vi "Chad Magic Voodoo 4.vi"() -> ()   [LabVIEW 2016]
panel:
  in  "Automatic Wire\n Feed not to Exceed":dbl=1.4
  in  "Add Wire Feed... (%)":dbl=4.0
  in  "For Every... (mm)":dbl=0.2
  out "W trigger Y":dbl
  out "C trigger Y":dbl
  out "R trigger Y":dbl
  in  "Window Bead Trigger heights":dbl[](array[numeric])
  in  "Robot Bead Trigger heights":dbl[](array[numeric])
  in  "Center Bead Trigger heights":dbl[](array[numeric])
  out "Shutter Open":bool
  in  "base path":path=path "C:/Users/Mark/Desktop/BeadScan"
  in  "Write Code":bool
  out "Bead3 Size":i32
  out "Bead2 Size":i32
  out "Bead1 Size":i32
  in  "Tab Control":T1(tab)
  in  "Mark Target Bead Height":bool
  out "All Beads":cluster{dbl[], dbl[]}[](graph)
  out "Target Bead Height":dbl
  in  "Set Correction C":bool
  in  "Set Trigger Offset":dbl
  in  "Center Bead Corrections":dbl[](array[numeric])
  in  "Center Bead Trigger Positions":dbl[](array[numeric])
  out "Center Bead #1":cluster{dbl[], dbl[]}[](graph)
  out "Center Bead Trigger":dbl
  in  "Set Trigger Center":bool
  in  "Undo":bool
  out "Difference From Bead Height Setpoint C":dbl
  out "Recommended % Change\n in Wire Feed C":dbl
  in  "Set Correction R":bool
  in  "Set Trigger Offset 2":dbl
  out "Robot Bead #2":cluster{dbl[], dbl[]}[](graph)
  in  "Robot Bead Trigger Positions":dbl[](array[numeric])
  in  "Robot Bead Corrections":dbl[](array[numeric])
  out "Robot Bead Trigger":dbl
  in  "Set Trigger Robot":bool
  in  "Undo":bool
  out "Difference From Bead Height Setpoint R":dbl
  out "Recommended % Change\n in Wire Feed R":dbl
  in  "Set Correction W":bool
  in  "Set Trigger Offset 3":dbl
  out "Window Bead #3":cluster{dbl[], dbl[]}[](graph)
  in  "Window Bead Trigger Positions":dbl[](array[numeric])
  in  "Window Bead Corrections":dbl[](array[numeric])
  out "Window Bead Trigger":dbl
  in  "Set Trigger Window":bool
  in  "Undo":bool
  out "Difference From Bead Height Setpoint W":dbl
  out "Recommended % Change\n in Wire Feed W":dbl
  in  "stop":bool
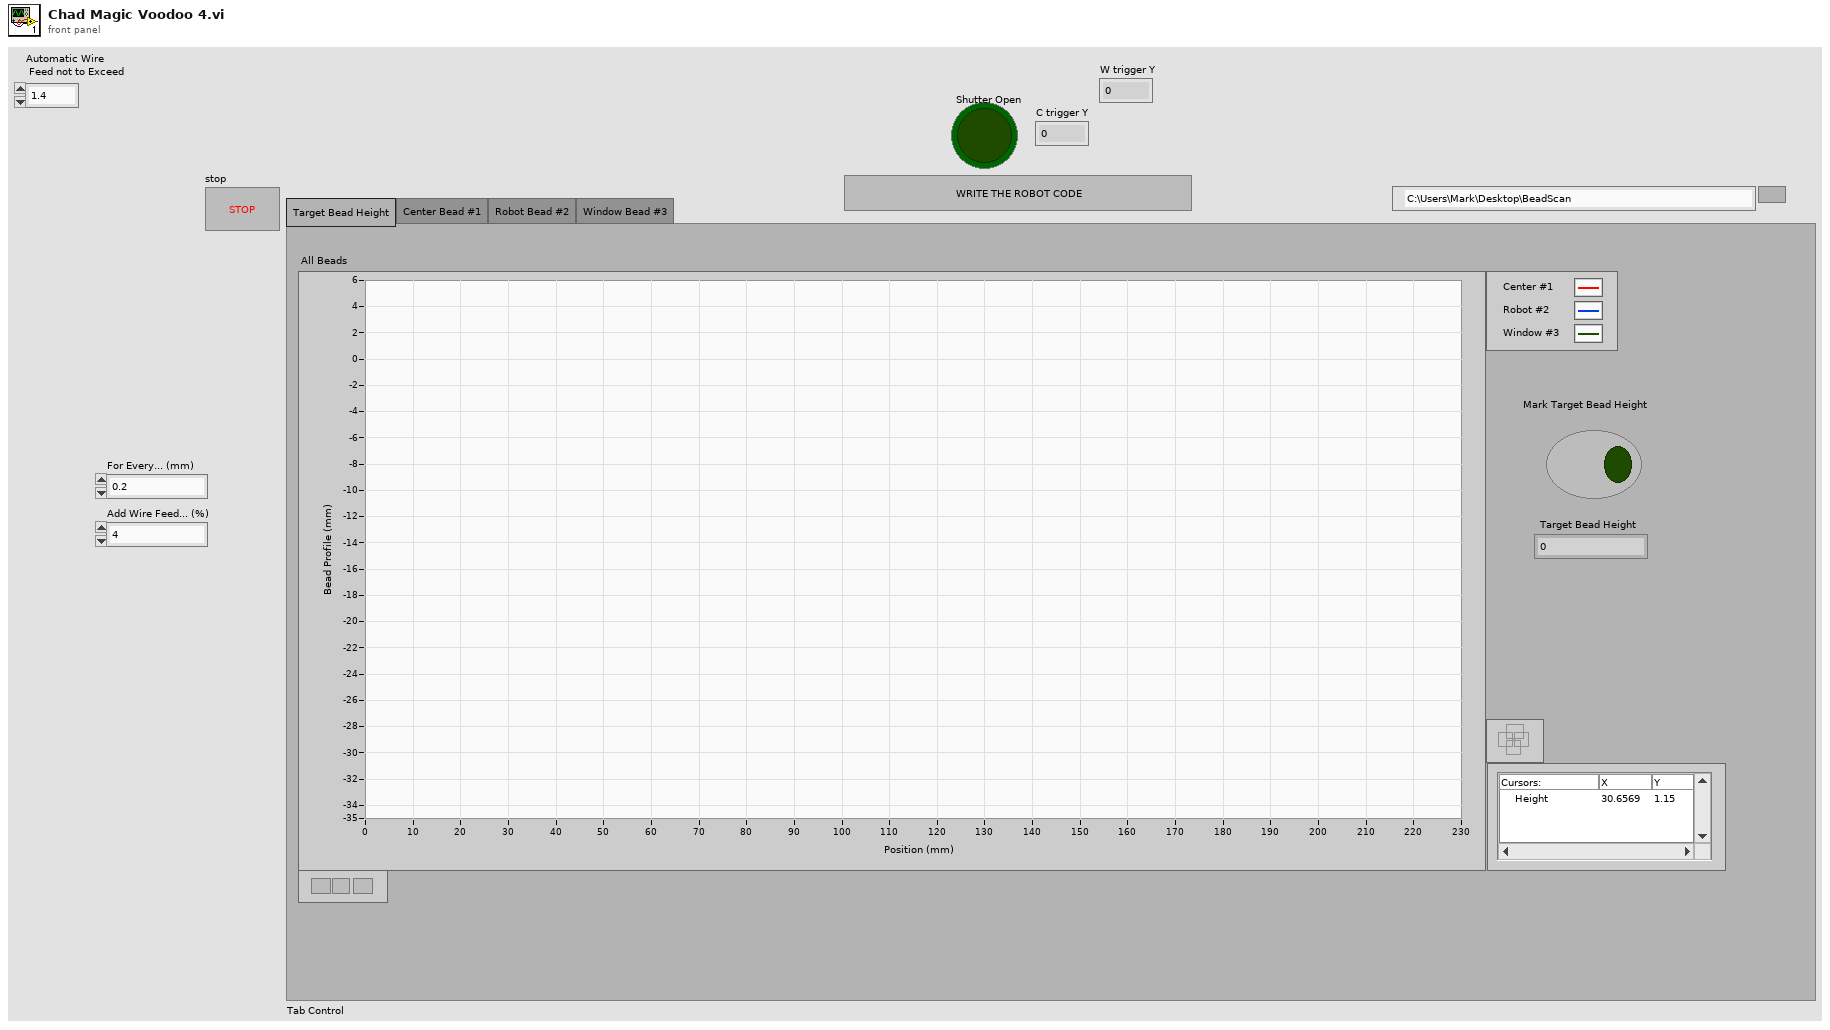
[diagram p1: front panel]
types:
  T1 = enum32{"Target Bead Height", "Center Bead #1", "Robot Bead #2", "Window Bead #3"}
  T2 = enum16{"open", "replace", "create", "open or create", "replace or create", "replace or create with confirmation"}
  T3 = cluster{"[0]":cluster{dbl[], dbl[]}, "[1]":cluster{dbl[], dbl[]}, "[2]":cluster{dbl[], dbl[]}}
  T4 = cluster{dbl[], "Center Bead Trigger heights":dbl[]}
  T5 = cluster{dbl[], "Window Bead Trigger heights":dbl[]}
  T6 = cluster{dbl[], "Robot Bead Trigger heights":dbl[]}
  T7 = cluster{dbl[], "Center Bead Trigger heights":dbl[]}[]
  T8 = cluster{dbl[], "Robot Bead Trigger heights":dbl[]}[]
  T9 = cluster{dbl[], "Window Bead Trigger heights":dbl[]}[]
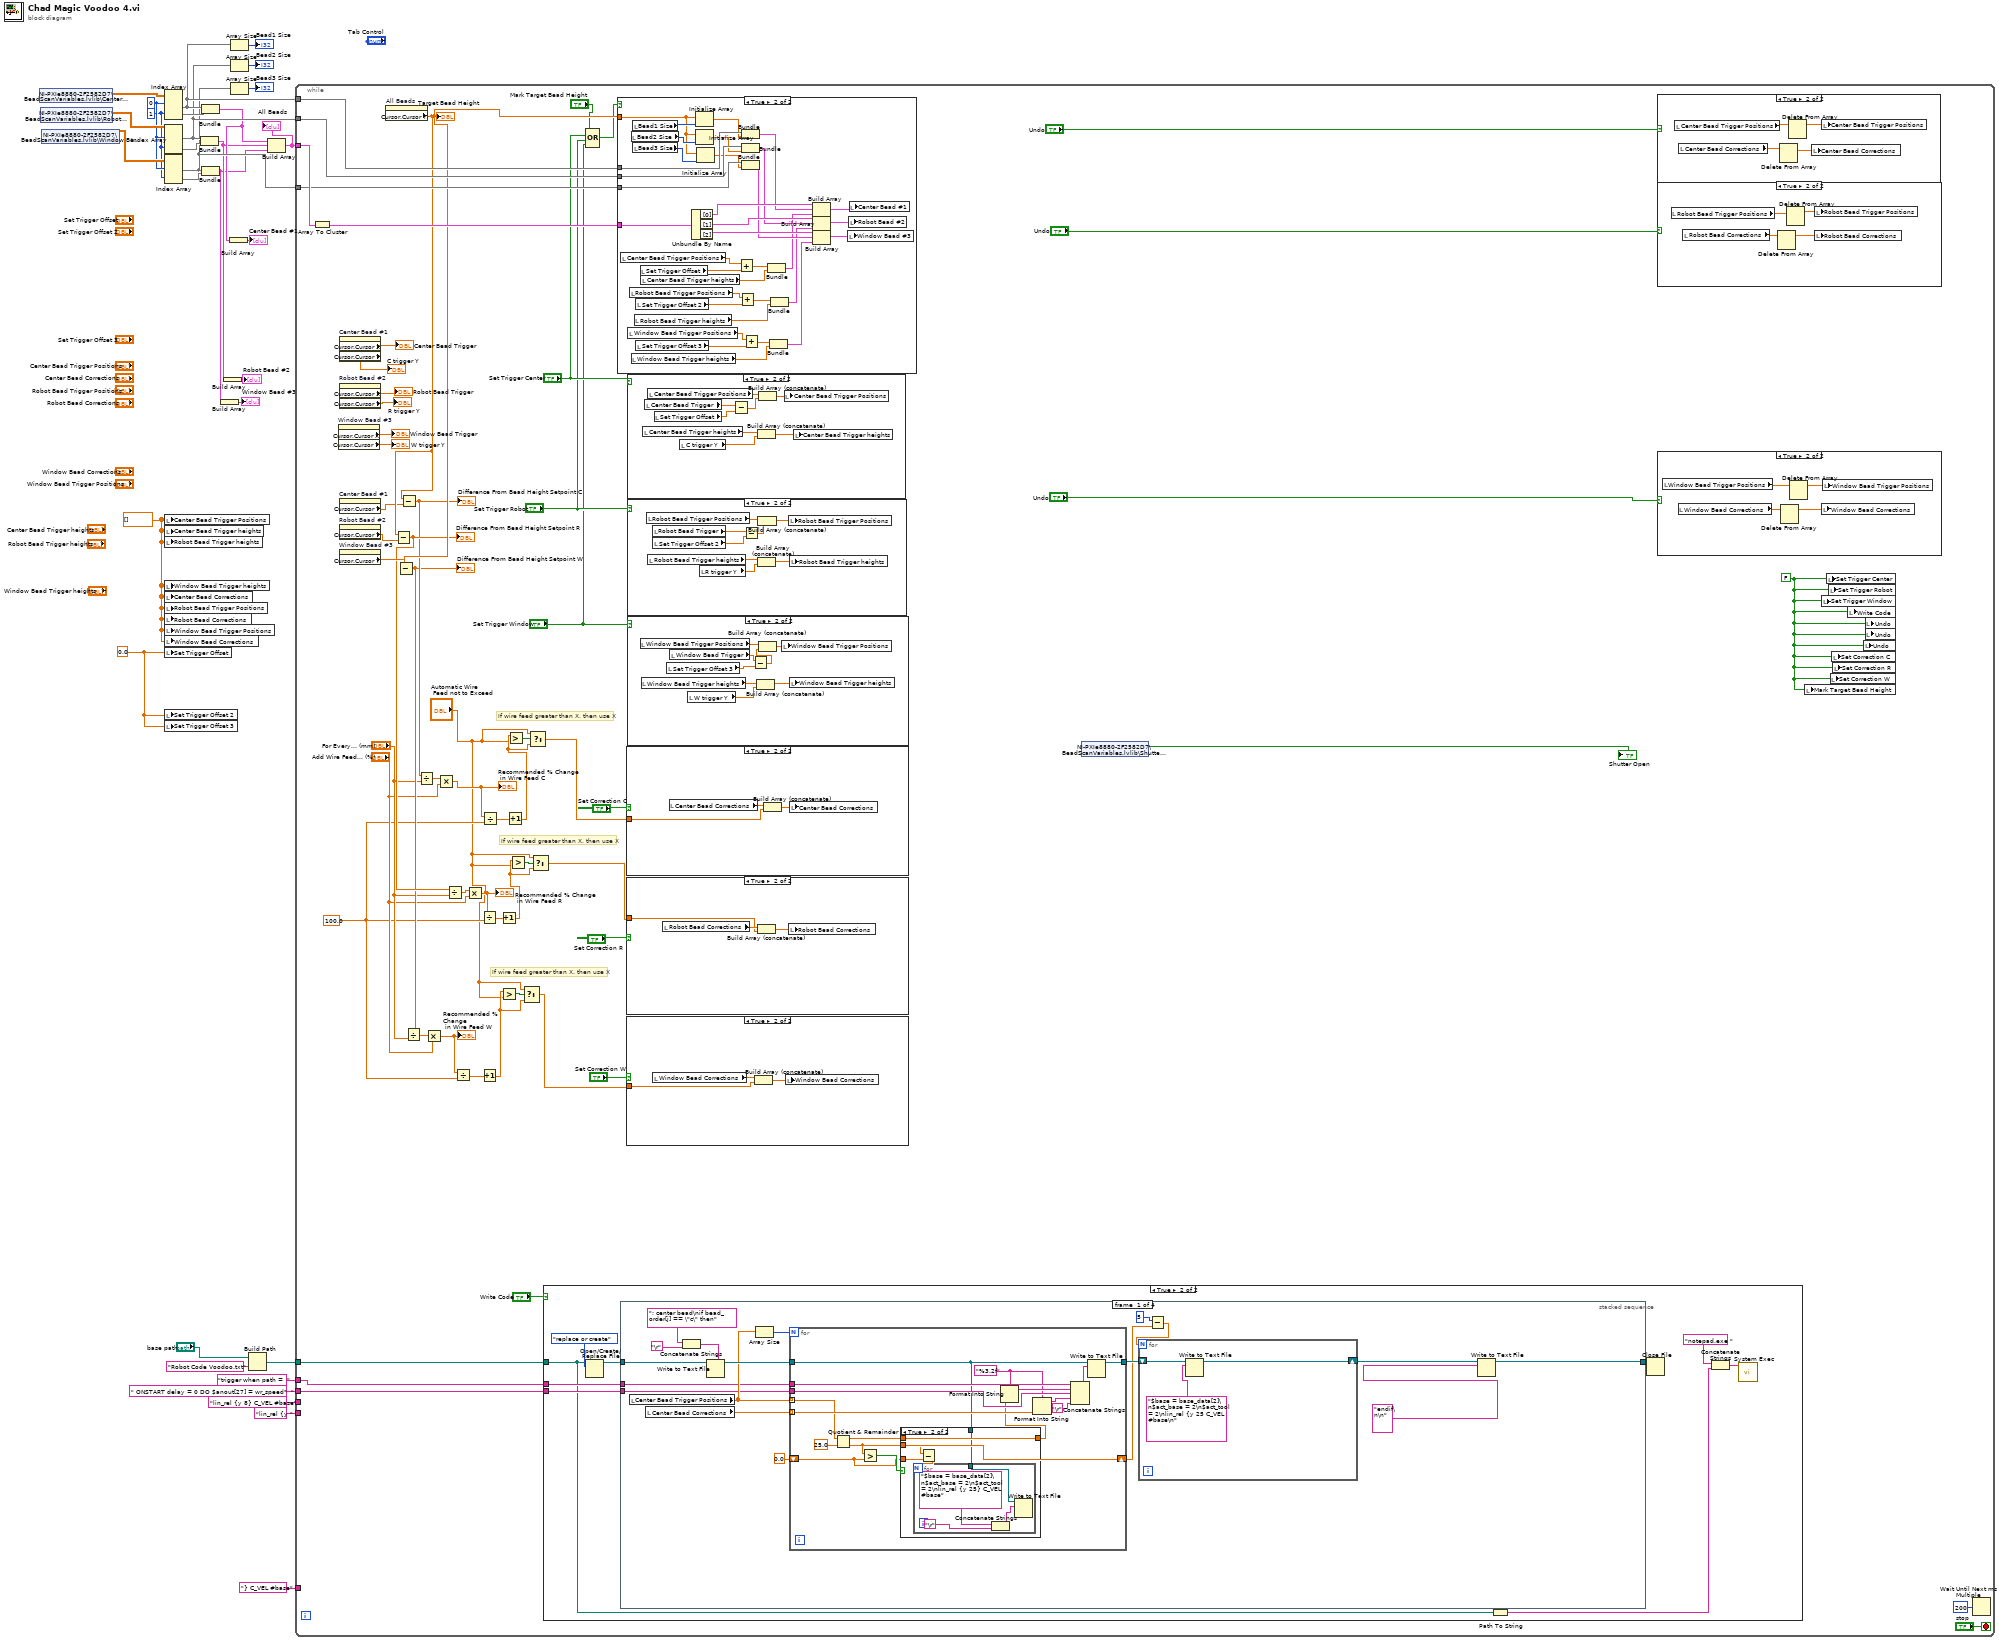
[diagram p0: block diagram]
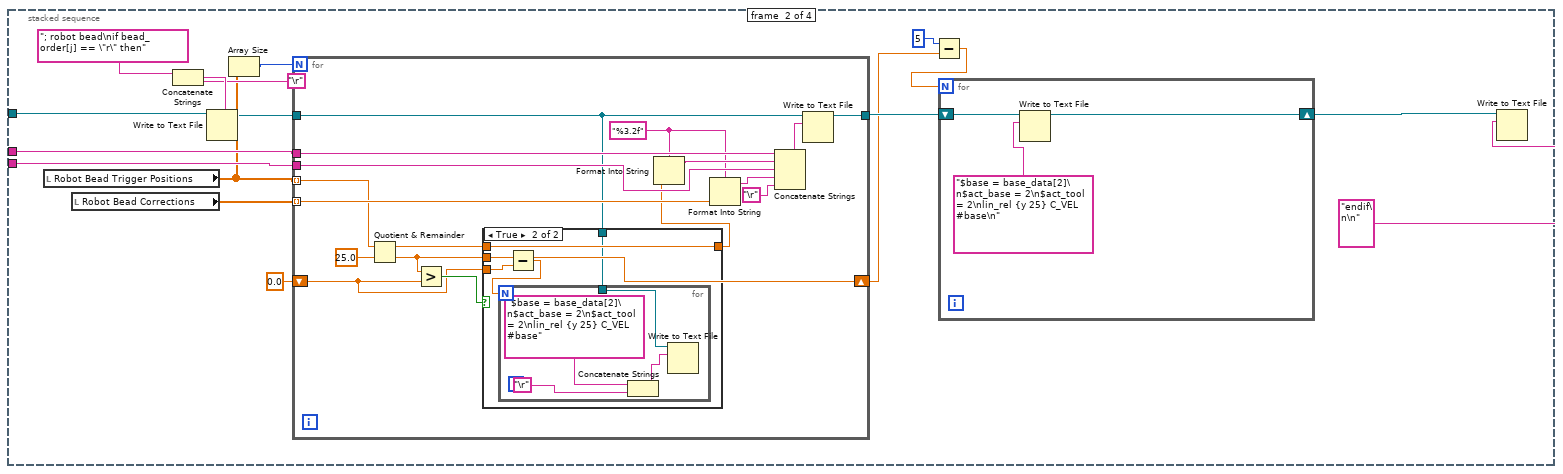
[diagram p7: hidden frame]
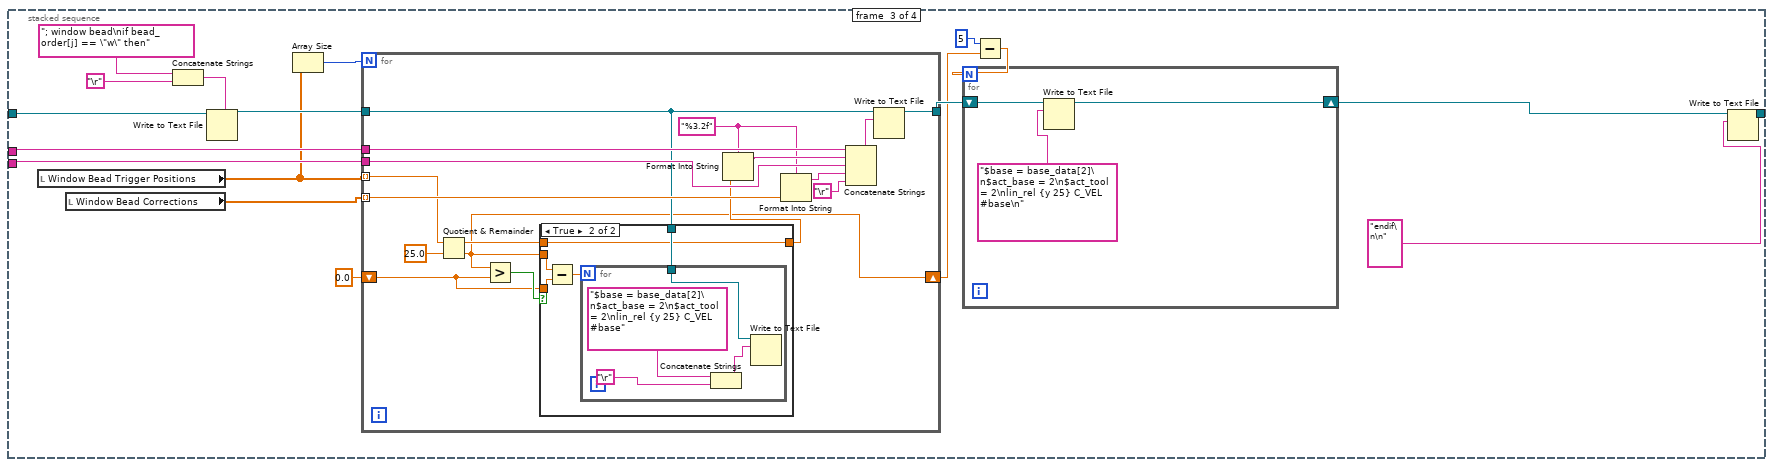
[diagram p9: hidden frame]
diagram:
  w2 = 0.0
  w1 = dbl[] []
  w26 = 1 ("index (row)")
  w27 = 0 ("index (row)")
  n1 = shared-variable "NI-PXIe8880-2F2582D7\\BeadScanVariables.lvlib\\Center Bead #1"() -> (w31:dbl[][])  [unwired: 1 in, 1 out]
  n2 = shared-variable "NI-PXIe8880-2F2582D7\\BeadScanVariables.lvlib\\Robot Bead #2"() -> (w29:dbl[][])  [unwired: 1 in, 1 out]
  n3 = shared-variable "NI-PXIe8880-2F2582D7\\BeadScanVariables.lvlib\\Window Bead #3"() -> (w28:dbl[][])  [unwired: 1 in, 1 out]
  n4 = Index Array(array=w31, index (row) #1=w27, index (row) #2=w26) -> (element #1=w19:dbl[], element #2=w30:dbl[])  [unwired: 2 in]
  n5 = Index Array(array=w29, index (row) #1=w27, index (row) #2=w26) -> (element #1=w18:dbl[], element #2=w25:dbl[])  [unwired: 2 in]
  n6 = Index Array(array=w28, index (row) #1=w27, index (row) #2=w26) -> (element #1=w17:dbl[], element #2=w24:dbl[])  [unwired: 2 in]
  n7 = local write "Center Bead Trigger Positions"(w1) -> ()
  n8 = local write "Center Bead Trigger heights"(w1) -> ()
  n9 = local write "Robot Bead Trigger heights"(w1) -> ()
  n10 = local write "Window Bead Trigger heights"(w1) -> ()
  n11 = local write "Center Bead Corrections"(w1) -> ()
  n12 = local write "Robot Bead Trigger Positions"(w1) -> ()
  n13 = local write "Robot Bead Corrections"(w1) -> ()
  n14 = local write "Window Bead Trigger Positions"(w1) -> ()
  n15 = local write "Window Bead Corrections"(w1) -> ()
  n16 = local write "Set Trigger Offset"(w2) -> ()
  n17 = local write "Set Trigger Offset 2"(w2) -> ()
  n18 = local write "Set Trigger Offset 3"(w2) -> ()
  n19 = Bundle(w18, w25) -> (w14:cluster{dbl[], dbl[]})  [unwired: 1 in]
  n20 = Bundle(w19, w30) -> (w15:cluster{dbl[], dbl[]})  [unwired: 1 in]
  n21 = Bundle(w17, w24) -> (w11:cluster{dbl[], dbl[]})  [unwired: 1 in]
  n22 = Build Array(w11) -> (→"Window Bead #3":cluster{dbl[], dbl[]}[])
  n23 = Build Array(w14) -> (→"Robot Bead #2":cluster{dbl[], dbl[]}[])
  n24 = Build Array(w15) -> (→"Center Bead #1":cluster{dbl[], dbl[]}[])
  n25 = Array Size(array=w19) -> (size(s)=→"Bead1 Size":i32)
  n26 = Array Size(array=w18) -> (size(s)=→"Bead2 Size":i32)
  n27 = Array Size(array=w17) -> (size(s)=→"Bead3 Size":i32)
  n28 = Build Path(base path="base path", name or relative path="Robot Code Voodoo.txt") -> (appended path=w8:path)
  n29 = Build Array(w15, w14, w11) -> (w20:cluster{dbl[], dbl[]}[])
  "All Beads" <- w20
  n30 = while {
    tunnel: w20 -> [w87]
    tunnel: w19 -> [w85]
    tunnel: w18 -> [w84]
    tunnel: w17 -> [w83]
    tunnel: w8 -> [w78]
    tunnel: "trigger when path =  " -> [w77]
    tunnel: " ONSTART delay = 0 DO $anout[27] = wr_speed*  " -> [w76]
    tunnel: "lin_rel {y 8} C_VEL #base" -> [_]
    tunnel: "lin_rel {y " -> [_]
    tunnel: "} C_VEL #base" -> [_]
    stop <- "stop" stop-if-true
    w46 = 100.0 ("y")
    w42 = FALSE
    # "If wire feed greater than X, then use X"
    # "If wire feed greater than X, then use X"
    # "If wire feed greater than X, then use X"
    n31 = Array To Cluster(array=w87) -> (cluster=w86:T3)
    n32 = property on="Window Bead #3" class="XYGraph (strict)"() -> ("Cursor.Cursor X"=→"Window Bead Trigger":dbl, "Cursor.Cursor Y"=→"W trigger Y":dbl)  [unwired: 2 in, 2 out]
    n33 = property on="Center Bead #1" class="XYGraph (strict)"() -> ("Cursor.Cursor X"=→"Center Bead Trigger":dbl, "Cursor.Cursor Y"=→"C trigger Y":dbl)  [unwired: 2 in, 2 out]
    n34 = property on="Robot Bead #2" class="XYGraph (strict)"() -> ("Cursor.Cursor X"=→"Robot Bead Trigger":dbl, "Cursor.Cursor Y"=→"R trigger Y":dbl)  [unwired: 2 in, 2 out]
    n35 = property on="Center Bead #1" class="XYGraph (strict)"() -> ("Cursor.Cursor Y"=w72:dbl)  [unwired: 2 in, 2 out]
    n36 = property on="Robot Bead #2" class="XYGraph (strict)"() -> ("Cursor.Cursor Y"=w71:dbl)  [unwired: 2 in, 2 out]
    n37 = property on="Window Bead #3" class="XYGraph (strict)"() -> ("Cursor.Cursor Y"=w70:dbl)  [unwired: 2 in, 2 out]
    n38 = property on="All Beads" class="XYGraph (strict)"() -> ("Cursor.Cursor Y"=w73:dbl)  [unwired: 2 in, 2 out]
    "Target Bead Height" <- w73
    n39 = Subtract(x=w73, y=w71) -> (x-y=w58:dbl)
    "Difference From Bead Height Setpoint R" <- w58
    n40 = Subtract(x=w73, y=w70) -> (x-y=w55:dbl)
    "Difference From Bead Height Setpoint W" <- w55
    n41 = Subtract(x=w73, y=w72) -> (x-y=w56:dbl)
    "Difference From Bead Height Setpoint C" <- w56
    n42 = Divide(x=w55, y="For Every... (mm)") -> (x/y=w59:dbl)
    n43 = Divide(x=w56, y="For Every... (mm)") -> (x/y=w57:dbl)
    n44 = Multiply(x=w59, y="Add Wire Feed... (%)") -> (x*y=w47:dbl)
    "Recommended % Change\n in Wire Feed W" <- w47
    n45 = Multiply(x=w57, y="Add Wire Feed... (%)") -> (x*y=w48:dbl)
    "Recommended % Change\n in Wire Feed C" <- w48
    n46 = Divide(x=w58, y="For Every... (mm)") -> (x/y=w60:dbl)
    n47 = Divide(x=w47, y=w46) -> (x/y=w43:dbl)
    n48 = Multiply(x=w60, y="Add Wire Feed... (%)") -> (x*y=w49:dbl)
    "Recommended % Change\n in Wire Feed R" <- w49
    n49 = Divide(x=w49, y=w46) -> (x/y=w45:dbl)
    n50 = Increment(x=w43) -> (x+1=w35:dbl)
    n51 = Divide(x=w48, y=w46) -> (x/y=w44:dbl)
    n52 = Increment(x=w45) -> (x+1=w33:dbl)
    n53 = Greater?(x=w35, y="Automatic Wire\n Feed not to Exceed") -> (0:w37:bool)
    n54 = Increment(x=w44) -> (x+1=w39:dbl)
    n55 = Greater?(x=w39, y="Automatic Wire\n Feed not to Exceed") -> (0:w41:bool)
    n56 = Greater?(x=w33, y="Automatic Wire\n Feed not to Exceed") -> (0:w38:bool)
    n57 = Select(t="Automatic Wire\n Feed not to Exceed", s=w37, f=w35) -> (s? t:f=w36:dbl)
    n58 = Select(t="Automatic Wire\n Feed not to Exceed", s=w41, f=w39) -> (s? t:f=w40:dbl)
    n59 = Select(t="Automatic Wire\n Feed not to Exceed", s=w38, f=w33) -> (s? t:f=w34:dbl)
    n60 = case shown="True" "Write Code" {
      tunnel: w78 -> [_ w100]
      tunnel: w77 -> [_ w107]
      tunnel: w76 -> [_ w106]
      frame False {
      }
      frame True {
        n61 = Open/Create/Replace File(file path (use dialog)=w100, operation (0:open)=T2."replace or create") -> (refnum out=w108:refnum<file>)  [unwired: 4 in, 2 out]
        n62 = stacked-sequence {
          tunnel: w108 -> [w123 w171 w218 _]
          tunnel: w107 -> [w118 w168 w213 _]
          tunnel: w106 -> [w117 w167 w212 _]
          tunnel: [w114 _ _ _] -> w105
          frame #0 {
            n63 = local read "Center Bead Trigger Positions"() -> (w120:dbl[])
            n64 = local read "Center Bead Corrections"() -> (w119:dbl[])
            n65 = Concatenate Strings("; center bead\nif bead_order[j] == \"c\" then", "\r") -> (w124:string)
            n66 = Write to Text File(file (use dialog)=w123, text=w124) -> (refnum out=w122:refnum<file>)  [unwired: 2 in, 2 out]
            n67 = Array Size(array=w120) -> (size(s)=w121:i32)
            n68 = for {
              N: w121 -> [_]
              tunnel: w122 -> [w132]
              tunnel: w120 -> [w137] mode=indexing
              tunnel: w119 -> [w142] mode=indexing
              tunnel: w118 -> [w146]
              tunnel: w117 -> [w143]
              tunnel: [w140] -> w115
              shift-right: [w131] -> w110
              shift-left: 0.0 -> [w130]
              w139 = "%3.2f" ("format string")
              n69 = Quotient & Remainder(x=w137, y=25.0) -> (x-y*floor(x/y)=w134:dbl, floor(x/y)=w131:dbl)
              n70 = Greater?(x=w131, y=w130) -> (0:w135:bool)
              n71 = case shown="True" w135 {
                tunnel: w134 -> [w147 w152]
                tunnel: [w147 w152] -> w133
                tunnel: w132 -> [_ w151]
                tunnel: w131 -> [_ w150]
                tunnel: w130 -> [_ w149]
                frame False {
                }
                frame True {
                  n72 = Subtract(x=w150, y=w149) -> (x-y=w148:dbl)
                  n73 = for {
                    N: w148 -> [_]
                    tunnel: w151 -> [w156]
                    n74 = Concatenate Strings("$base = base_data[2]\n$act_base = 2\n$act_tool = 2\nlin_rel {y 25} C_VEL #base", "\r") -> (w153:string)
                    n75 = Write to Text File(file (use dialog)=w156, text=w153) -> ()  [unwired: 2 in, 3 out]
                  }
                }
              }
              n76 = Format Into String(format string=w139, w133) -> (resulting string=w145:string)  [unwired: 2 in, 1 out]
              n77 = Format Into String(format string=w139, w142) -> (resulting string=w141:string)  [unwired: 2 in, 1 out]
              n78 = Concatenate Strings(w146, w145, w143, w141, "\r") -> (w144:string)
              n79 = Write to Text File(file (use dialog)=w132, text=w144) -> (refnum out=w140:refnum<file>)  [unwired: 2 in, 2 out]
            }
            n80 = Subtract(x=5, y=w110) -> (x-y=w109:dbl)
            n81 = for {
              N: w109 -> [_]
              shift-right: [w127] -> w113
              shift-left: w115 -> [w129]
              n82 = Write to Text File(file (use dialog)=w129, text="$base = base_data[2]\n$act_base = 2\n$act_tool = 2\nlin_rel {y 25 C_VEL #base\n") -> (refnum out=w127:refnum<file>)  [unwired: 2 in, 2 out]
            }
            n83 = Write to Text File(file (use dialog)=w113, text="endif\n\n") -> (refnum out=w114:refnum<file>)  [unwired: 2 in, 2 out]
          }
          frame #1 {
            n84 = local read "Robot Bead Trigger Positions"() -> (w166:dbl[])
            n85 = local read "Robot Bead Corrections"() -> (w165:dbl[])
            n86 = Concatenate Strings("; robot bead\nif bead_order[j] == \"r\" then", "\r") -> (w172:string)
            n87 = Write to Text File(file (use dialog)=w171, text=w172) -> (refnum out=w164:refnum<file>)  [unwired: 2 in, 2 out]
            n88 = Array Size(array=w166) -> (size(s)=w163:i32)
            n89 = for {
              N: w163 -> [_]
              tunnel: w164 -> [w179]
              tunnel: w166 -> [w184] mode=indexing
              tunnel: w165 -> [w189] mode=indexing
              tunnel: w168 -> [w193]
              tunnel: w167 -> [w190]
              tunnel: [w187] -> w158
              shift-right: [w178] -> w157
              shift-left: 0.0 -> [w177]
              w186 = "%3.2f" ("format string")
              n90 = Quotient & Remainder(x=w184, y=25.0) -> (x-y*floor(x/y)=w181:dbl, floor(x/y)=w178:dbl)
              n91 = Greater?(x=w178, y=w177) -> (0:w182:bool)
              n92 = case shown="True" w182 {
                tunnel: w181 -> [w194 w199]
                tunnel: [w194 w199] -> w180
                tunnel: w179 -> [_ w198]
                tunnel: w178 -> [_ w197]
                tunnel: w177 -> [_ w196]
                frame False {
                }
                frame True {
                  n93 = Subtract(x=w197, y=w196) -> (x-y=w195:dbl)
                  n94 = for {
                    N: w195 -> [_]
                    tunnel: w198 -> [w203]
                    n95 = Concatenate Strings("$base = base_data[2]\n$act_base = 2\n$act_tool = 2\nlin_rel {y 25} C_VEL #base", "\r") -> (w200:string)
                    n96 = Write to Text File(file (use dialog)=w203, text=w200) -> ()  [unwired: 2 in, 3 out]
                  }
                }
              }
              n97 = Format Into String(format string=w186, w180) -> (resulting string=w192:string)  [unwired: 2 in, 1 out]
              n98 = Format Into String(format string=w186, w189) -> (resulting string=w188:string)  [unwired: 2 in, 1 out]
              n99 = Concatenate Strings(w193, w192, w190, w188, "\r") -> (w191:string)
              n100 = Write to Text File(file (use dialog)=w179, text=w191) -> (refnum out=w187:refnum<file>)  [unwired: 2 in, 2 out]
            }
            n101 = Subtract(x=5, y=w157) -> (x-y=w159:dbl)
            n102 = for {
              N: w159 -> [_]
              shift-right: [w174] -> w162
              shift-left: w158 -> [w176]
              n103 = Write to Text File(file (use dialog)=w176, text="$base = base_data[2]\n$act_base = 2\n$act_tool = 2\nlin_rel {y 25} C_VEL #base\n") -> (refnum out=w174:refnum<file>)  [unwired: 2 in, 2 out]
            }
            n104 = Write to Text File(file (use dialog)=w162, text="endif\n\n") -> ()  [unwired: 2 in, 3 out]
          }
          frame #2 {
            n105 = local read "Window Bead Trigger Positions"() -> (w211:dbl[])
            n106 = local read "Window Bead Corrections"() -> (w210:dbl[])
            n107 = Concatenate Strings("; window bead\nif bead_order[j] == \"w\" then", "\r") -> (w219:string)
            n108 = Write to Text File(file (use dialog)=w218, text=w219) -> (refnum out=w214:refnum<file>)  [unwired: 2 in, 2 out]
            n109 = Array Size(array=w211) -> (size(s)=w215:i32)
            n110 = for {
              N: w215 -> [_]
              tunnel: w214 -> [w226]
              tunnel: w211 -> [w231] mode=indexing
              tunnel: w210 -> [w236] mode=indexing
              tunnel: w213 -> [w240]
              tunnel: w212 -> [w237]
              tunnel: [w234] -> w205
              shift-right: [w225] -> w204
              shift-left: 0.0 -> [w224]
              w233 = "%3.2f" ("format string")
              n111 = Quotient & Remainder(x=w231, y=25.0) -> (x-y*floor(x/y)=w228:dbl, floor(x/y)=w225:dbl)
              n112 = Greater?(x=w225, y=w224) -> (0:w229:bool)
              n113 = case shown="True" w229 {
                tunnel: w228 -> [w241 w245]
                tunnel: [w241 w245] -> w227
                tunnel: w226 -> [_ w246]
                tunnel: w225 -> [_ w243]
                tunnel: w224 -> [_ w242]
                frame False {
                }
                frame True {
                  n114 = Subtract(x=w243, y=w242) -> (x-y=w244:dbl)
                  n115 = for {
                    N: w244 -> [_]
                    tunnel: w246 -> [w250]
                    n116 = Concatenate Strings("$base = base_data[2]\n$act_base = 2\n$act_tool = 2\nlin_rel {y 25} C_VEL #base", "\r") -> (w247:string)
                    n117 = Write to Text File(file (use dialog)=w250, text=w247) -> ()  [unwired: 2 in, 3 out]
                  }
                }
              }
              n118 = Format Into String(format string=w233, w227) -> (resulting string=w239:string)  [unwired: 2 in, 1 out]
              n119 = Format Into String(format string=w233, w236) -> (resulting string=w235:string)  [unwired: 2 in, 1 out]
              n120 = Concatenate Strings(w240, w239, w237, w235, "\r") -> (w238:string)
              n121 = Write to Text File(file (use dialog)=w226, text=w238) -> (refnum out=w234:refnum<file>)  [unwired: 2 in, 2 out]
            }
            n122 = Subtract(x=5, y=w204) -> (x-y=w206:dbl)
            n123 = for {
              N: w206 -> [_]
              shift-right: [w221] -> w209
              shift-left: w205 -> [w223]
              n124 = Write to Text File(file (use dialog)=w223, text="$base = base_data[2]\n$act_base = 2\n$act_tool = 2\nlin_rel {y 25} C_VEL #base\n") -> (refnum out=w221:refnum<file>)  [unwired: 2 in, 2 out]
            }
            n125 = Write to Text File(file (use dialog)=w209, text="endif\n\n") -> ()  [unwired: 2 in, 3 out]
          }
          frame #3 {
          }
        }
        n126 = Path To String(path=w100) -> (string=w101:string)
        n127 = Close File(refnum=w105) -> ()  [unwired: 1 in, 2 out]
        n128 = Concatenate Strings("notepad.exe " ("command line"), w101) -> (w103:string)
        n129 = call <vilib>:"System Exec.vi"("command line"=w103) -> ()  [unwired: 7 in, 4 out]
      }
    }
    n130 = Compound Arithmetic op=OR("Mark Target Bead Height", "Set Trigger Center", "Set Trigger Robot", "Set Trigger Window") -> (w64:bool)
    n131 = case shown="True" w64 {
      tunnel: w73 -> [_ w319]
      tunnel: w86 -> [_ w317]
      tunnel: w85 -> [_ w316]
      tunnel: w84 -> [_ w314]
      tunnel: w83 -> [_ w313]
      frame False {
      }
      frame True {
        n132 = local read "Center Bead Trigger Positions"() -> (w297:dbl[])
        n133 = local read "Window Bead Trigger Positions"() -> (w291:dbl[])
        n134 = local read "Robot Bead Trigger Positions"() -> (w294:dbl[])
        n135 = local read "Bead2 Size"() -> (w320:i32)
        n136 = local read "Window Bead Trigger heights"() -> (w290:dbl[])
        n137 = local read "Bead1 Size"() -> (w321:i32)
        n138 = local read "Bead3 Size"() -> (w318:i32)
        n139 = local read "Robot Bead Trigger heights"() -> (w292:dbl[])
        n140 = local read "Set Trigger Offset 2"() -> (w300:dbl)
        n141 = local read "Set Trigger Offset 3"() -> (w299:dbl)
        n142 = local read "Set Trigger Offset"() -> (w301:dbl)
        n143 = local read "Center Bead Trigger heights"() -> (w295:dbl[])
        n144 = Unbundle By Name(w317) -> ("[0]"=w310:cluster{dbl[], dbl[]}, "[1]"=w308:cluster{dbl[], dbl[]}, "[2]"=w306:cluster{dbl[], dbl[]})
        n145 = Initialize Array(w319, w321) -> (w315:dbl[])
        n146 = Initialize Array(w319, w320) -> (w311:dbl[])
        n147 = Initialize Array(w319, w318) -> (w312:dbl[])
        n148 = Add(x=w297, y=w301) -> (x+y=w296:dbl[])
        n149 = Add(x=w294, y=w300) -> (x+y=w293:dbl[])
        n150 = Bundle(w316, w315) -> (w309:cluster{dbl[], dbl[]})  [unwired: 1 in]
        n151 = Bundle(w314, w311) -> (w307:cluster{dbl[], dbl[]})  [unwired: 1 in]
        n152 = Bundle(w313, w312) -> (w305:cluster{dbl[], dbl[]})  [unwired: 1 in]
        n153 = Add(x=w291, y=w299) -> (x+y=w298:dbl[])
        n154 = Bundle(w296, "Center Bead Trigger heights"=w295) -> (w289:T4)  [unwired: 1 in]
        n155 = Bundle(w298, "Window Bead Trigger heights"=w290) -> (w287:T5)  [unwired: 1 in]
        n156 = Bundle(w293, "Robot Bead Trigger heights"=w292) -> (w288:T6)  [unwired: 1 in]
        n157 = Build Array(w310, w309, w289) -> (w304:T7)
        n158 = Build Array(w308, w307, w288) -> (w303:T8)
        n159 = Build Array(w306, w305, w287) -> (w302:T9)
        n160 = local write "Window Bead #3"(w302) -> ()
        n161 = local write "Robot Bead #2"(w303) -> ()
        n162 = local write "Center Bead #1"(w304) -> ()
      }
    }
    n163 = case shown="True" "Set Correction C" {
      tunnel: w40 -> [_ w97]
      frame False {
      }
      frame True {
        n164 = local read "Center Bead Corrections"() -> (w99:dbl[])
        n165 = Build Array (concatenate)(w99, w97) -> (w98:dbl[])
        n166 = local write "Center Bead Corrections"(w98) -> ()
      }
    }
    n167 = case shown="True" "Set Correction R" {
      tunnel: w34 -> [_ w94]
      frame False {
      }
      frame True {
        n168 = local read "Robot Bead Corrections"() -> (w96:dbl[])
        n169 = Build Array (concatenate)(w96, w94) -> (w95:dbl[])
        n170 = local write "Robot Bead Corrections"(w95) -> ()
      }
    }
    n171 = case shown="True" "Set Correction W" {
      tunnel: w36 -> [_ w91]
      frame False {
      }
      frame True {
        n172 = local read "Window Bead Corrections"() -> (w93:dbl[])
        n173 = Build Array (concatenate)(w93, w91) -> (w92:dbl[])
        n174 = local write "Window Bead Corrections"(w92) -> ()
      }
    }
    n175 = case shown="True" "Set Trigger Center" {
      frame False {
      }
      frame True {
        n176 = local read "Center Bead Trigger heights"() -> (w281:dbl[])
        n177 = local read "Center Bead Trigger"() -> (w284:dbl)
        n178 = local read "Center Bead Trigger Positions"() -> (w286:dbl[])
        n179 = local read "Set Trigger Offset"() -> (w282:dbl)
        n180 = local read "C trigger Y"() -> (w280:dbl)
        n181 = Subtract(x=w284, y=w282) -> (x-y=w283:dbl)
        n182 = Build Array (concatenate)(w281, w280) -> (w279:dbl[])
        n183 = Build Array (concatenate)(w286, w283) -> (w285:dbl[])
        n184 = local write "Center Bead Trigger Positions"(w285) -> ()
        n185 = local write "Center Bead Trigger heights"(w279) -> ()
      }
    }
    n186 = case shown="True" "Set Trigger Robot" {
      frame False {
      }
      frame True {
        n187 = local read "Robot Bead Trigger Positions"() -> (w278:dbl[])
        n188 = local read "Robot Bead Trigger heights"() -> (w272:dbl[])
        n189 = local read "Robot Bead Trigger"() -> (w276:dbl)
        n190 = local read "Set Trigger Offset 2"() -> (w274:dbl)
        n191 = local read "R trigger Y"() -> (w271:dbl)
        n192 = Subtract(x=w276, y=w274) -> (x-y=w275:dbl)
        n193 = Build Array (concatenate)(w272, w271) -> (w273:dbl[])
        n194 = Build Array (concatenate)(w278, w275) -> (w277:dbl[])
        n195 = local write "Robot Bead Trigger Positions"(w277) -> ()
        n196 = local write "Robot Bead Trigger heights"(w273) -> ()
      }
    }
    n197 = case shown="True" "Set Trigger Window" {
      frame False {
      }
      frame True {
        n198 = local read "Window Bead Trigger Positions"() -> (w270:dbl[])
        n199 = local read "Window Bead Trigger heights"() -> (w265:dbl[])
        n200 = local read "Set Trigger Offset 3"() -> (w268:dbl)
        n201 = local read "Window Bead Trigger"() -> (w267:dbl)
        n202 = local read "W trigger Y"() -> (w264:dbl)
        n203 = Subtract(x=w267, y=w268) -> (x-y=w266:dbl)
        n204 = Build Array (concatenate)(w265, w264) -> (w263:dbl[])
        n205 = Build Array (concatenate)(w270, w266) -> (w269:dbl[])
        n206 = local write "Window Bead Trigger Positions"(w269) -> ()
        n207 = local write "Window Bead Trigger heights"(w263) -> ()
      }
    }
    n208 = shared-variable "NI-PXIe8880-2F2582D7\\BeadScanVariables.lvlib\\Shutter Open"() -> (→"Shutter Open":bool)  [unwired: 1 in, 1 out]
    n209 = case shown="True" "Undo" {
      frame False {
      }
      frame True {
        n210 = local read "Robot Bead Trigger Positions"() -> (w257:dbl[])
        n211 = local read "Robot Bead Corrections"() -> (w258:dbl[])
        n212 = Delete From Array(array=w258) -> (array with subset deleted=w255:dbl[])  [unwired: 2 in, 1 out]
        n213 = Delete From Array(array=w257) -> (array with subset deleted=w256:dbl[])  [unwired: 2 in, 1 out]
        n214 = local write "Robot Bead Trigger Positions"(w256) -> ()
        n215 = local write "Robot Bead Corrections"(w255) -> ()
      }
    }
    n216 = case shown="True" "Undo" {
      frame False {
      }
      frame True {
        n217 = local read "Window Bead Trigger Positions"() -> (w253:dbl[])
        n218 = local read "Window Bead Corrections"() -> (w252:dbl[])
        n219 = Delete From Array(array=w252) -> (array with subset deleted=w251:dbl[])  [unwired: 2 in, 1 out]
        n220 = Delete From Array(array=w253) -> (array with subset deleted=w254:dbl[])  [unwired: 2 in, 1 out]
        n221 = local write "Window Bead Corrections"(w251) -> ()
        n222 = local write "Window Bead Trigger Positions"(w254) -> ()
      }
    }
    n223 = case shown="True" "Undo" {
      frame False {
      }
      frame True {
        n224 = local read "Center Bead Trigger Positions"() -> (w261:dbl[])
        n225 = local read "Center Bead Corrections"() -> (w260:dbl[])
        n226 = Delete From Array(array=w260) -> (array with subset deleted=w259:dbl[])  [unwired: 2 in, 1 out]
        n227 = Delete From Array(array=w261) -> (array with subset deleted=w262:dbl[])  [unwired: 2 in, 1 out]
        n228 = local write "Center Bead Corrections"(w259) -> ()
        n229 = local write "Center Bead Trigger Positions"(w262) -> ()
      }
    }
    n230 = local write "Mark Target Bead Height"(w42) -> ()
    n231 = local write "Set Trigger Window"(w42) -> ()
    n232 = local write "Set Trigger Center"(w42) -> ()
    n233 = local write "Set Trigger Robot"(w42) -> ()
    n234 = local write "Set Correction W"(w42) -> ()
    n235 = local write "Set Correction C"(w42) -> ()
    n236 = local write "Set Correction R"(w42) -> ()
    n237 = local write "Write Code"(w42) -> ()
    n238 = local write "Undo"(w42) -> ()
    n239 = local write "Undo"(w42) -> ()
    n240 = local write "Undo"(w42) -> ()
    n241 = Wait Until Next ms Multiple(millisecond multiple=u32 200) -> ()  [unwired: 1 out]
  }
